vi "Constants.vi"() -> ()   [LabVIEW 2018, in "NI-XNET Monitor Shared.lvlib"]
doc: "Use this Global VI to access the GUIDs assigned to the page resources of the Custom Device."
uses:
  NI-XNET Monitor Shared.lvlib
panel:
  in  "Tab Control":enum32{"GUIDS", "Constants", "Properties"}(tab)=enum."Properties"
  in  "NIVS.Native.XNET.LIN.disabled":string="2e183a89-6016-4f90-b470-f06827b093be-DISABLED"
  in  "NIVS.Native.XNET.FlexRay.disabled":string="2cc91995-c247-480b-a96d-47b20600b52a-DISABLED"
  in  "NIVS.Native.XNET.CAN.disabled":string="389a82a6-36c1-4557-a906-147449b05d6a-DISABLED"
  in  "NIVS.Native.XNET.LIN":string="2e183a89-6016-4f90-b470-f06827b093be"
  in  "NIVS.Native.XNET.FlexRay":string="2cc91995-c247-480b-a96d-47b20600b52a"
  in  "NIVS.Native.XNET.CAN":string="389a82a6-36c1-4557-a906-147449b05d6a"
  in  "NIVS.Native.XNET":string="6b693e6d-67b1-40b8-8108-4a4cc3147721"
  in  "Interface LIN":string="c19a2e81-5516-4045-93a5-b1bca7ac20ae"
  in  "Interface FlexRay":string="b3b15e68-7151-4c2d-a280-06a82878b967"
  in  "PortError":string="37c19a15-61f7-4078-98c8-bfb7f6b25de3"
  in  "PortStatus":string="20dbf2c1-039f-4944-a9cd-53b00268baa8"
  in  "Interface CAN":string="d0ed4327-8d71-4af7-8daf-159d159a2198"
  in  "Port":string="6e4b4e9f-3d48-4140-aa73-eb1a9ddd4810"
  in  "NI-XNET Monitor":string="2fba45b0-1589-4179-a966-5fc49498794e"
  in  "CD.RT.Init.Msg":string="Async NI-XNET Monitoring Custom Device Starting....\n"
  in  "PortError.Name":string="Error"
  in  "PortStatus.Name":string="Status"
  in  "CD.Main.Description":string="This is an asynchronous Custom Device which allows you to open parallel sessions to an existing NI-XNET ports and allows you to monitor port condition."
  in  "BusLoad.Period":string="BusLoad.Period"
  in  "BusLoad.Disable":string="BusLoad.Disable"
  in  "Referenced.XNET.Port.Path":string="Referenced.XNET.Port.Path"
  in  "NI-XNET.Port.IO.Name":string="NI-XNET.Port.IO.Name"
  in  "Force.Disable.Port.Mon":string="Force.Disable.Port.Mon"
  in  "Referenced.XNET.Port":string="Referenced.XNET.Port"
  in  "Compiled.Settings":string="Compiled.Settings"
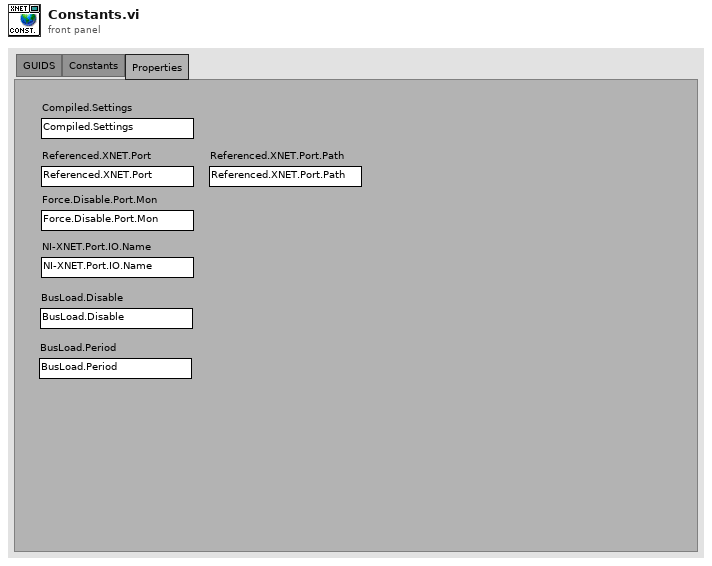
[diagram p1: front panel]
diagram:
